vi "To String.vi"(11 "JSON Datatype in":refnum<class "JSON Datatype.lvclass">) -> (2 "String":string)   [LabVIEW 2017, in "LVJSON.lvlib" / "JSON Datatype.lvclass"]
uses:
  JSON Datatype.lvclass
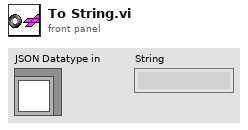
[diagram p1: front panel]
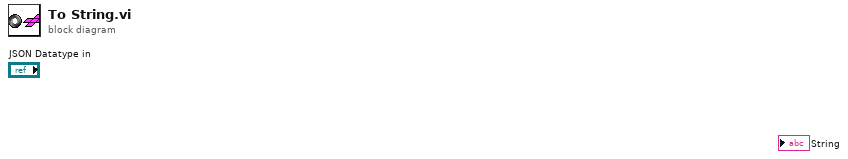
[diagram p0: block diagram]
diagram:
